vi "CryoCon Calibration Tables.vi"() -> ()   [LabVIEW 2020]
uses:
  Sub Controls/CryoCon Sensor Type.ctl
panel:
  in  "Voltage Bias":T1(ring)=enum."3 mV"
  in  "Sensor Type":T2=enum."DC Resistance 625 ½"
  in  "stop":bool
  out "Scale Factor":dbl[](array[numeric]) format="%.2f"
  out "Type":T2[](array[typedef])
  in  "delete":bool
  in  "add":bool
  in  "User Calibrations":i32[](listbox)
  out "Names":string[](array[string])
  in  "VISA session":refnum<visa-resource-name>
  # "Set Sensor Type and\nexcitation for curve to\nbe loaded, then press \"Add\""
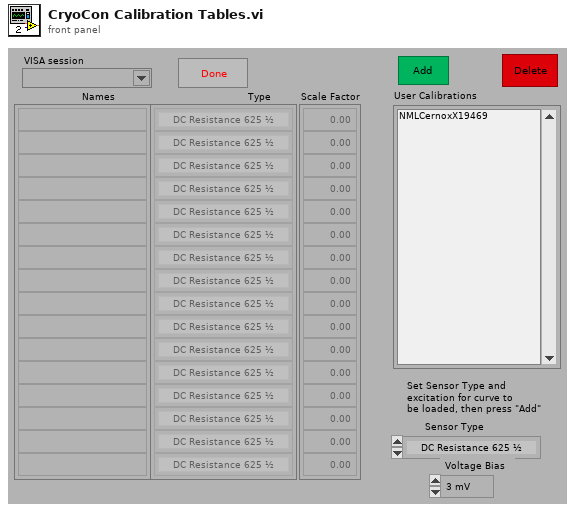
[diagram p1: front panel]
types:
  T1 = enum16{"10 mV", "3 mV", "1 mV", "320 uV", "100 uV", "32 uV", "10 uV"}
  T2 = typedef "CryoCon Sensor Type.ctl" = enum16{"Diode", "AC Resistance", "DC Resistance 3.1 k½", "DC Resistance 312 ½", "DC Resistance 625 ½"}
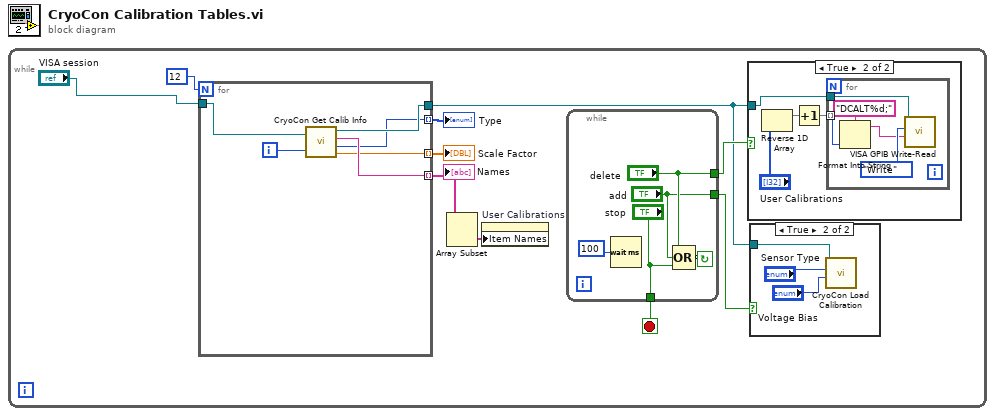
[diagram p0: block diagram]
diagram:
  n1 = while {
    stop <- w5 stop-if-true
    n2 = for {
      N: 12 -> [_]
      tunnel: "VISA session" -> [w33]
      tunnel: [w30] -> w8 mode=indexing
      tunnel: [w29] -> w10 mode=indexing
      tunnel: [w32] -> w4
      tunnel: [w28] -> w1 mode=indexing
      i -> [w31]
      n3 = call "CryoCon Get Calib Info.vi"("VISA session"=w33, "Index"=w31) -> ("dup VISA session"=w32:refnum<visa-resource-name>, "Sensor Name"=w30:string, "Sensor Type 2"=w28:T2, "Multiplier"=w29:dbl)  [unwired: 2 in]
    }
    "Names" <- w8
    "Type" <- w1
    "Scale Factor" <- w10
    n4 = Array Subset(array=w8) -> (w9:string[])  [unwired: 2 in]
    n5 = property on="User Calibrations" class="LstBox (strict)"("Item Names"=w9) -> ()  [unwired: 2 in, 2 out]
    n6 = while {
      tunnel: ["stop"] -> w5
      tunnel: ["add"] -> w6
      tunnel: ["delete"] -> w7
      stop <- w14 continue-if-true
      n7 = Wait (ms)(milliseconds to wait=u32 100) -> ()  [unwired: 1 out]
      n8 = Compound Arithmetic op=OR("delete", "add", "stop") -> (invert w14:bool)
    }
    n9 = case shown="True" w7 {
      tunnel: w4 -> [_ w20]
      frame False {
      }
      frame True {
        n10 = Reverse 1D Array(array="User Calibrations") -> (reversed array=w19:i32[])
        n11 = Increment(x=w19) -> (x+1=w22:i32[])
        n12 = for {
          tunnel: w22 -> [w26] mode=indexing
          tunnel: w20 -> [w25]
          n13 = Format Into String(format string="DCALT%d;" ("Format String"), w26) -> (resulting string=w23:string)  [unwired: 2 in, 1 out]
          n14 = call "VISA GPIB Write-Read.vi"("Command"=w23, "Action"=enum16{"Write", "Read", "Write & Read"}."Write", "VISA resource name"=w25) -> ()  [unwired: 5 in, 4 out]
        }
      }
    }
    n15 = case shown="True" w6 {
      tunnel: w4 -> [_ w16]
      frame False {
      }
      frame True {
        n16 = call "CryoCon Load Calibration.vi"("Instrument Address"=w16, "Sensor Type"="Sensor Type", "Sensor Number"="Voltage Bias") -> ()  [unwired: 3 in, 3 out]
      }
    }
  }
